vi "ztscopeM Trigger Video.vi"(4 "Line":i32=1, 5 "Standard":i32(ring)=1 items=["PAL", "NTSC", "SECAM"], 6 "Field":i32=1, 7 "Level Mode":i32(ring)=1 items=["Auto", "Manual"], 8 "error in":errorcluster, 9 "Level":dbl, 10 "Source":i32(ring)=10 items=["TTL0", "TTL1", "TTL2", "TTL3", "TTL4", "TTL5", "TTL6", "TTL7", "ECL0", "ECL1", "Input Channel 1", "Input Channel 2", "Input Channel 3", "Input Channel 4", "External Trigger Source", "STAR", "Manual Trigger", "Pattern"], 11 "Instrument Handle In":i32) -> (0 "error out":errorcluster, 3 "Instrument Handle Out":i32)   [LabVIEW 2011]
doc: "Set the instrument to trigger on video and configure the video trigger settings."
uses:
  ztscopeM.dll
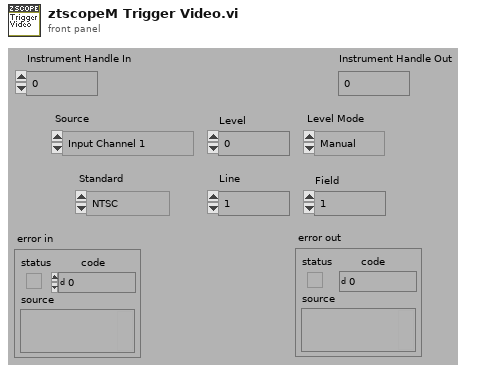
[diagram p1: front panel]
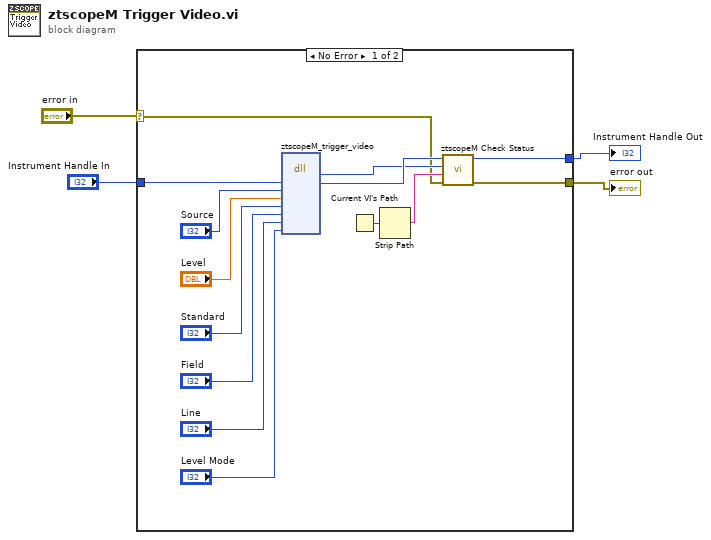
[diagram p0: block diagram]
diagram:
  n1 = case shown="No Error" "error in" {
    selector: "error in" -> [w7 w20]
    tunnel: [w6 w20] -> w1
    tunnel: "Instrument Handle In" -> [w18 w19]
    tunnel: [w5 w19] -> w2
    frame No Error {
      n2 = dll-call lib="C:/Program Files/National Instruments/LabVIEW 2011/instr.lib/ztscopem/ztscopeM.dll" fn="ztscopeM_trigger_video"("instrumentHandle"=w18, "source"="Source", "level"="Level", "standard"="Standard", "field"="Field", "line"="Line", "levelMode"="Level Mode") -> (w8:i32, "instrumentHandle"=w9:i32)  [unwired: 9 in, 2 out]
      n3 = Current VI's Path() -> (path=w11:path)
      n4 = Strip Path(path=w11) -> (name=w10:string)  [unwired: 1 out]
      n5 = call "ztscopeM Check Status.vi"("error in"=w7, "name of VI"=w10, "status"=w8, "instrument handle in"=w9) -> ("error out"=w6:errorcluster, "instrument handle out"=w5:i32)  [unwired: 2 in]
    }
    frame Error {
    }
  }
  "Instrument Handle Out" <- w2
  "error out" <- w1
